vi "Timeout.vi"(1 "Timeout":u32, 2 "Initialize":bool) -> (0 "Timed Out?":bool)   [LabVIEW 2020]
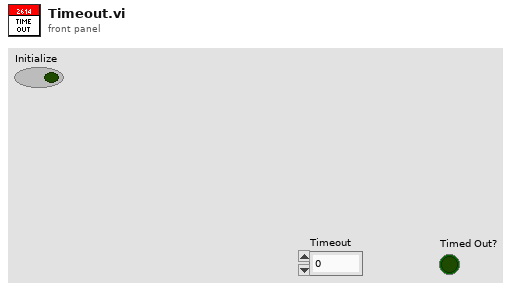
[diagram p1: front panel]
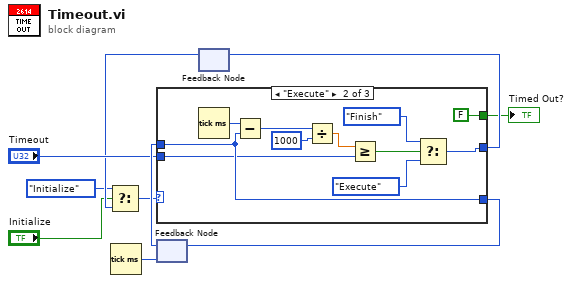
[diagram p0: block diagram]
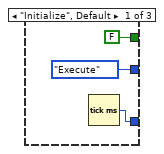
[diagram p2: hidden frame]
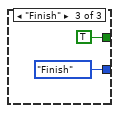
[diagram p3: hidden frame]
diagram:
  n1 = Tick Count (ms)() -> (millisecond timer value=w6:u32)
  n2 = feedback #1(w6) -> (w8:u32)
  n3 = feedback #2() -> (w4:enum16{"Initialize", "Execute", "Finish"})  [unwired: 1 in]
  n4 = Select(t=enum16{"Initialize", "Execute", "Finish"}."Initialize", s="Initialize", f=w4) -> (s? t:f=w3:enum16{"Initialize", "Execute", "Finish"})
  n5 = case shown="\"Execute\"" w3 {
    tunnel: [enum16{"Initialize", "Execute", "Finish"}."Execute" w24 enum16{"Initialize", "Execute", "Finish"}."Finish" ("t")] -> w10
    tunnel: [w13 w20 _] -> w9
    tunnel: w8 -> [_ w20 _]
    tunnel: "Timeout" -> [_ w18 _]
    tunnel: [FALSE FALSE TRUE] -> w5
    frame "Initialize", Default {
      n6 = Tick Count (ms)() -> (millisecond timer value=w13:u32)
    }
    frame "Execute" {
      n7 = Tick Count (ms)() -> (millisecond timer value=w21:u32)
      n8 = Subtract(x=w21, y=w20) -> (x-y=w17:u32)
      n9 = Divide(x=w17, y=u32 1000) -> (x/y=w15:dbl)
      n10 = Greater Or Equal?(x=w15, y=w18) -> (x >= y?=w19:bool)
      n11 = Select(t=enum16{"Initialize", "Execute", "Finish"}."Finish", s=w19, f=enum16{"Initialize", "Execute", "Finish"}."Execute" ("t")) -> (s? t:f=w24:enum16{"Initialize", "Execute", "Finish"})
    }
    frame "Finish" {
    }
  }
  "Timed Out?" <- w5
  n12 = feedback-in #1(w9) -> ()
  n13 = feedback-in #2(w10) -> ()
